vi "Build Target Map.vi"(8 "error in (no error)":errorcluster, 10 "Cluster in":refnum<class "Cluster.lvclass">) -> (0 "error out":errorcluster, 2 "Target Groups":map{string, T1}(c390))   [LabVIEW 2020, in "VolatusConfig.lvlib" / "Node.lvclass"]
uses:
  Node.lvclass
  Node.lvclass/Node.ctl
  Cluster/Cluster.lvclass
  lv-vecto/Vecto/Node Name ID.ctl
  lv-vecto/Vecto/Vecto.lvlib
  lv-vecto/VectoConfig/Target Group Info.ctl
  lv-vecto/VectoConfig/VectoConfig.lvlib
  VolatusConfigElement/VolatusConfigElement.lvclass
  C:/dev/lv20CE/relink/lv-volatus/VolatusConfig/VolatusConfigElement/VolatusConfigElement.lvclass
  C:/dev/lv20CE/relink/lv-volatus/VolatusConfig/Node/Node.lvclass
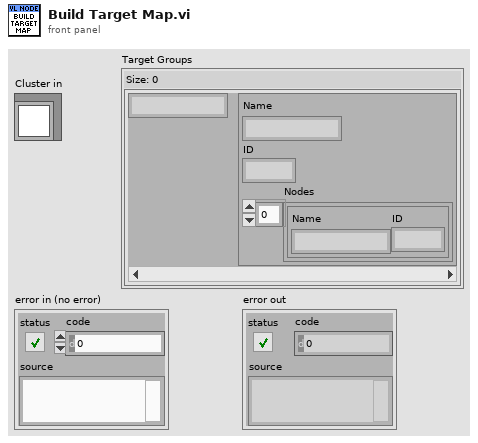
[diagram p1: front panel]
types:
  T1 = typedef "VectoConfig.lvlib/Target Group Info.ctl" = cluster{"Name":string, "ID":u32, "Nodes":T2[]}
  T2 = typedef "Vecto.lvlib/Node Name ID.ctl" = cluster{"Name":string, "ID":u32}
  T3 = typedef "VolatusConfig.lvlib/Target Group.ctl" = cluster{"Name":string, "ID":u32}
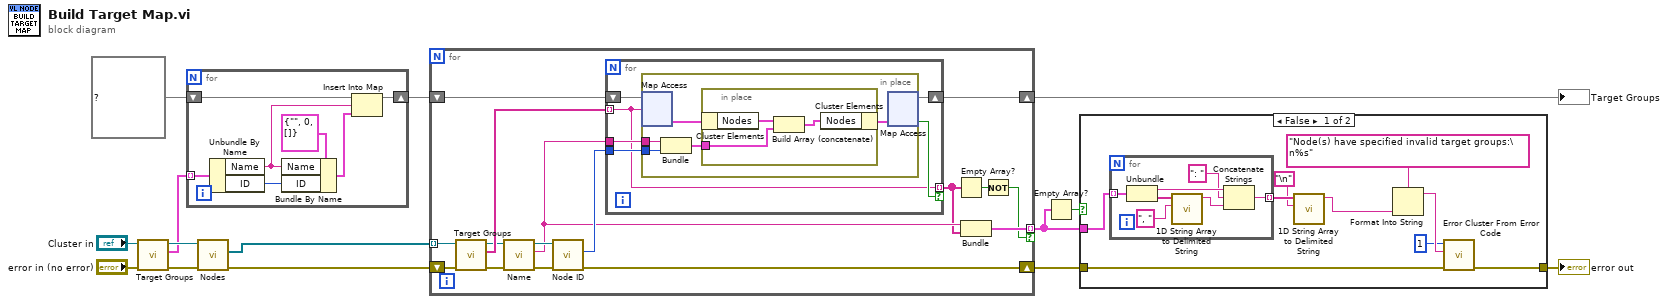
[diagram p0: block diagram]
diagram:
  n1 = call "Target Groups.vi"("error in (no error)"="error in (no error)", "Cluster in"="Cluster in") -> ("error out"=w12:errorcluster, "Target Groups"=w9:T3[], "Cluster out"=w13:refnum<class "Cluster.lvclass">)  [unwired: 7 in]
  n2 = for {
    shift-right: [w15] -> w8
    shift-left: map{string, T1} {} ("Target Groups") -> [w18]
    tunnel: w9 -> [w21] mode=indexing
    n3 = Unbundle By Name(w21) -> ("Name"=w16:string, "ID"=w19:u32)
    n4 = Bundle By Name(cluster=T1 {"Name"="", "ID"=0, "Nodes"=[]} ("Target Group Info"), "Name"=w16, "ID"=w19) -> (w17:T1)
    n5 = Insert Into Map(map in=w18, key=w16, value=w17) -> (map out=w15:map{string, T1})  [unwired: 2 out]
  }
  n6 = call "Nodes.vi"("error in (no error)"=w12, "Cluster in"=w13) -> ("error out"=w6:errorcluster, "Nodes"=w7:refnum<class "Node.lvclass">[])  [unwired: 7 in, 1 out]
  n7 = for {
    shift-right: [w28] -> w5
    shift-left: w8 -> [w34]
    tunnel: w7 -> [w36] mode=indexing
    shift-right: [w27] -> w4
    shift-left: w6 -> [w37]
    tunnel: [w23] -> w1 mode=indexing if=w22
    n8 = call "Target Groups.vi"("error in (no error)"=w37, "Node in"=w36) -> ("error out"=w33:errorcluster, "Target Groups"=w35:string[], "Node out"=w30:refnum<class "Node.lvclass">)  [unwired: 7 in]
    n9 = call "Name.vi"("error in (no error)"=w33, "VolatusConfigElement in"=w30) -> ("error out"=w31:errorcluster, "Name"=w26:string, "VolatusConfigElement out"=w29:refnum<class "Node.lvclass">)  [unwired: 7 in]
    n10 = call "Node ID.vi"("error in (no error)"=w31, "Node in"=w29) -> ("error out"=w27:errorcluster, "Node ID"=w32:u32)  [unwired: 7 in, 1 out]
    n11 = for {
      tunnel: w35 -> [w38] mode=indexing
      tunnel: w32 -> [w39]
      tunnel: w26 -> [w40]
      shift-right: [w41] -> w28
      shift-left: w34 -> [w43]
      tunnel: [w38] -> w25 mode=indexing if=w42
      n12 = in-place {
        in-place-border: w40 -> [w48]
        in-place-border: w39 -> [w47]
        n13 = in-place-map #1(w43, w38) -> (w46:T1)  [unwired: 1 in, 1 out]
        n14 = Bundle("Name"=w48, "Node ID"=w47) -> (w45:cluster{"Name":string, "Node ID":u32})  [unwired: 1 in]
        n15 = in-place {
          in-place-border: w45 -> [w50]
          n16 = in-place-cluster #2(w46) -> ("Nodes"=w51:T2[])
          n17 = Build Array (concatenate)(w51, w50) -> (w49:T2[])
          n18 = in-place-cluster #2("Nodes"=w49) -> (w44:T1)
        }
        n19 = in-place-map #1(w44) -> (w41:map{string, T1}, w42:bool)  [unwired: 1 in, 1 out]
      }
    }
    n20 = Empty Array?(array=w25) -> (empty?=w24:bool)
    n21 = Bundle("Name"=w26, w25) -> (w23:cluster{"Name":string, string[]})  [unwired: 1 in]
    n22 = Not(x=w24) -> (.not. x?=w22:bool)
  }
  "Target Groups" <- w5
  n23 = Empty Array?(array=w1) -> (empty?=w3:bool)
  n24 = case shown="False" w3 {
    tunnel: w4 -> [w55 w68]
    tunnel: [w54 w68] -> w2
    tunnel: w1 -> [w60 _]
    frame False {
      n25 = for {
        tunnel: w60 -> [w67] mode=indexing
        tunnel: [w61] -> w59 mode=indexing
        n26 = Unbundle(w67) -> ("Name"=w64:string, w66:string[])
        n27 = call <vilib>:"1D String Array to Delimited String.vi"("delimiter"=", ", "string array"=w66) -> ("delimited string"=w62:string)  [unwired: 9 in]
        n28 = Concatenate Strings(w64, ": " ("string"), w62) -> (w61:string)
      }
      n29 = call <vilib>:"1D String Array to Delimited String.vi"("delimiter"="\n", "string array"=w59) -> ("delimited string"=w56:string)  [unwired: 9 in]
      n30 = Format Into String(format string="Node(s) have specified invalid target groups:\n%s", w56) -> (resulting string=w53:string)  [unwired: 2 in, 1 out]
      n31 = call <vilib>:"Error Cluster From Error Code.vi"("error in (no error)"=w55, "error message (\"\")"=w53, "error code (0)"=1) -> ("error out"=w54:errorcluster)  [unwired: 6 in]
    }
    frame True {
    }
  }
  "error out" <- w2
